vi "Bump_Counter.vi"(0 "ref":dbl, 2 "cntrl":dbl, 3 "quanta":dbl, 4 "reset":bool) -> (5 "out":dbl)   [LabVIEW 2015]
uses:
  <vilib>/Rock Robotics/WPI/Joystick/WPI_JoystickDeviceEnum.ctl
  <vilib>/Rock Robotics/WPI/Joystick/WPI_JoystickAxis.ctl
panel:
  out "Out":dbl
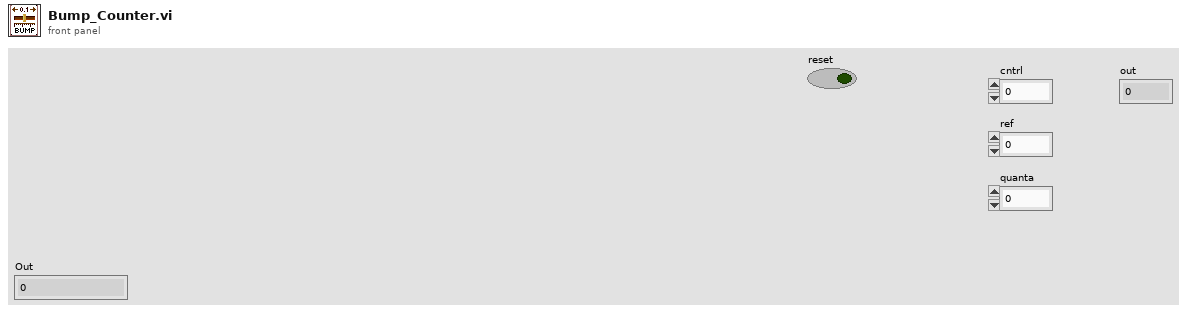
[diagram p1: front panel]
types:
  T1 = typedef "WPI_JoystickAxis.ctl" = enum16{"Axis 0", "Axis 1", "Axis 2", "Axis 3", "Axis 4", "Axis 5"}
  T2 = typedef "WPI_JoystickDevRef.ctl" = cluster{"Device":T3}
  T3 = typedef "WPI_JoystickDeviceEnum.ctl" = enum16{"USB 0", "USB 1", "USB 2", "USB 3", "USB 4", "USB 5"}
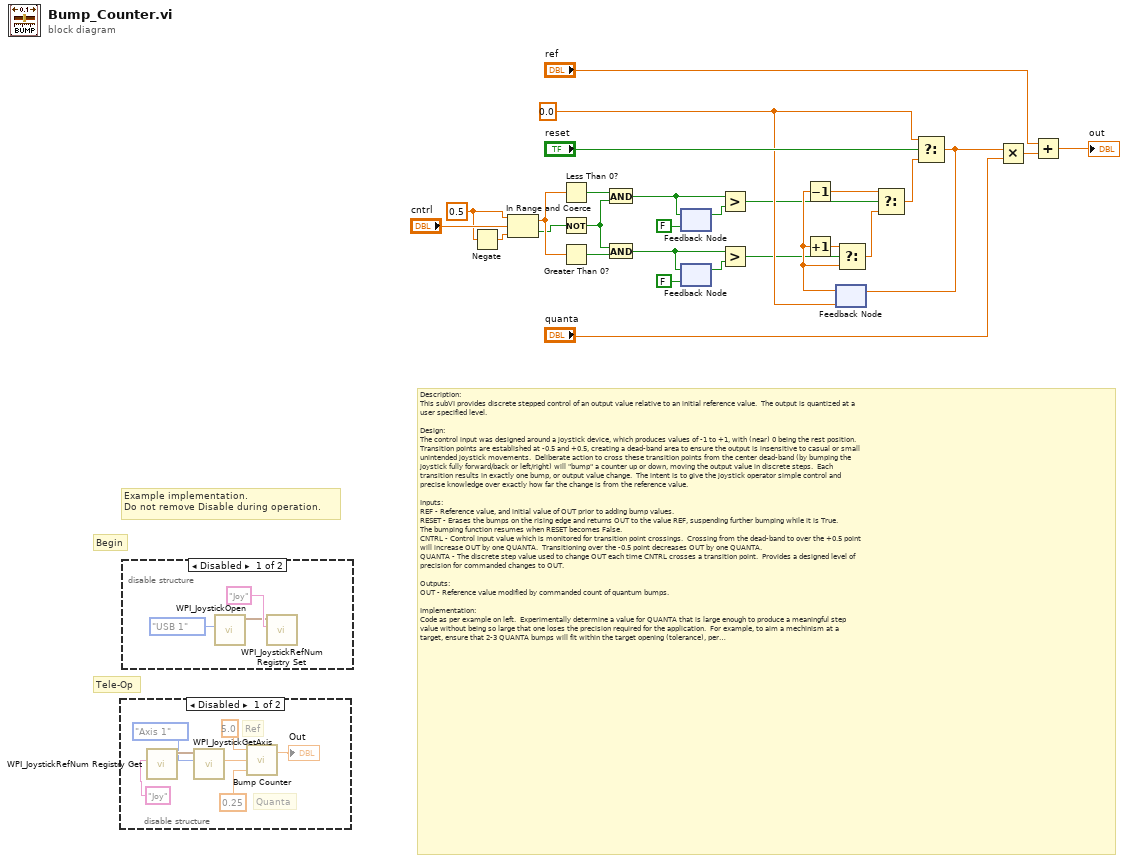
[diagram p0: block diagram]
diagram:
  w4 = 0.0 ("initial")
  w12 = 0.5 ("upper limit")
  # "Begin"
  # "Tele-Op"
  # "Example implementation.\nDo not remove Disable during operation."
  # "Description:\nThis subVI provides discrete stepped control of an output value relative to an initial reference value.  The output is quantized at a \nuser specified level.\n\nDesign:\nThe control input was designed around a joystick device, which produces values of -1 to +1, with (near) 0 being the rest position.  \nTransition points are established at -0.5 and +0.5, creating a dead-band area to ensure the output is insensitive to casual or small\nunintended joystick movements.  Deliberate action to cross these transition points from the center dead-band (by bumping the\njoystick fully forward/back or left/right) will \"bump\" a counter up or down, moving the output value in discrete steps.  Each \ntransition results in exactly one bump, or output value change.  The intent is to give the joystick operator simple control and \nprecise knowledge over exactly how far the change is from the reference value.\n\nInputs:\nREF - Reference value, and initial value of OUT prior to adding bump values.\nRESET - Erases the bumps on the rising edge and returns OUT to the value REF, suspending further bumping while it is True.\nThe bumping function resumes when RESET becomes False.\nCNTRL - Control input value which is monitored for transition point crossings.  Crossing from the dead-band to over the +0.5 point \nwill increase OUT by one QUANTA.  Transitioning over the -0.5 point decreases OUT by one QUANTA.\nQUANTA - The discrete step value used to change OUT each time CNTRL crosses a transition point.  Provides a designed level of\nprecision for commanded changes to OUT.\n\nOutputs:\nOUT - Reference value modified by commanded count of quantum bumps. \n\nImplementation:\nCode as per example on left.  Experimentally determine a value for QUANTA that is large enough to produce a meaningful step \nvalue without being so large that one loses the precision required for the application.  For example, to aim a mechinism at a \ntarget, ensure that 2-3 QUANTA bumps will fit within the target opening (tolerance), perhaps at low, mid, and high positions \nwithin the opening ... however, don't make QUANTA so small that it takes 'all day' to make an adjustment!\n\n----- RoboBees Team 836! -----  You too can change things ... consider a career in STEM!"
  n1 = disable-structure shown="Disabled" {
    frame Disabled {
      # "Ref"
      # "Quanta"
      n2 = call <vilib>:"WPI_JoystickRefNum Registry Get.vi"("refnum name"="Joy") -> ("JoystickDevRef"=w33:T2)  [unwired: 9 in, 1 out]
      n3 = call <vilib>:"WPI_JoystickGetAxis.vi"("Axis"=WPI_JoystickAxis."Axis 1", "JoystickDevRef"=w33) -> ("Value"=w31:dbl)  [unwired: 8 in, 1 out]
      n4 = call <userlib>:"Bump Counter.vi"("ref"=5.0, "cntrl"=w31, "quanta"=0.25) -> ("out"=→"Out":dbl)  [unwired: 3 in]
    }
    frame Enabled {
    }
  }
  n5 = disable-structure shown="Disabled" {
    frame Disabled {
      n6 = call <vilib>:"WPI_JoystickOpen.vi"("JoystickDevice"=WPI_JoystickDeviceEnum."USB 1") -> ("JoystickDevRef"=w37:T2)  [unwired: 10 in]
      n7 = call <vilib>:"WPI_JoystickRefNum Registry Set.vi"("refnum name"="Joy", "JoystickDevRef"=w37) -> ()  [unwired: 8 in, 2 out]
    }
    frame Enabled {
    }
  }
  n8 = Negate(x=w12) -> (-x=w13:dbl)
  n9 = In Range and Coerce(upper limit=w12, x="cntrl", lower limit=w13) -> (coerced(x)=w11:dbl, In Range?=w9:bool)
  n10 = Less Than 0?(x=w11) -> (x < 0?=w10:bool)
  n11 = Not(x=w9) -> (.not. x?=w7:bool)
  n12 = Greater Than 0?(x=w11) -> (x > 0?=w8:bool)
  n13 = And(x=w10, y=w7) -> (x .and. y?=w6:bool)
  n14 = And(x=w7, y=w8) -> (x .and. y?=w5:bool)
  n15 = feedback #1(FALSE ("down")) -> (w25:bool)
  n16 = feedback-in #1(w6) -> ()
  n17 = feedback #2(FALSE ("down")) -> (w22:bool)
  n18 = feedback-in #2(w5) -> ()
  n19 = Greater?(x=w6, y=w25) -> (0:w2:bool)
  n20 = Greater?(x=w5, y=w22) -> (0:w1:bool)
  n21 = feedback #3(w4) -> (w20:dbl)
  n22 = Decrement(x=w20) -> (x-1=w27:dbl)
  n23 = Increment(x=w20) -> (x+1=w26:dbl)
  n24 = Select(t=w26, s=w1, f=w20) -> (s? t:f=w28:dbl)
  n25 = Select(t=w27, s=w2, f=w28) -> (s? t:f=w19:dbl)
  n26 = Select(t=w4, s="reset", f=w19) -> (s? t:f=w3:dbl)
  n27 = feedback-in #3(w3) -> ()
  n28 = Multiply(x=w3, y="quanta") -> (x*y=w17:dbl)
  n29 = Add(x="ref", y=w17) -> (x+y=→"out":dbl)
